vi "NameToData.vi"(11 "Name":string) -> (3 "Target":T1)   [LabVIEW 2018]
uses:
  TargetDataType.ctl
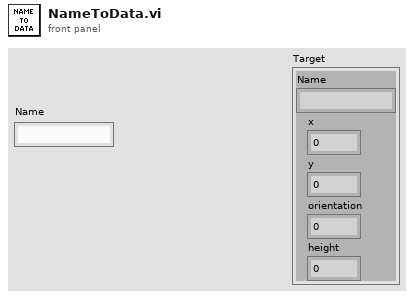
[diagram p1: front panel]
types:
  T1 = typedef "TargetDataType.ctl" = cluster{"Name":string, "x":dbl, "y":dbl, "orientation":dbl, "height":dbl}
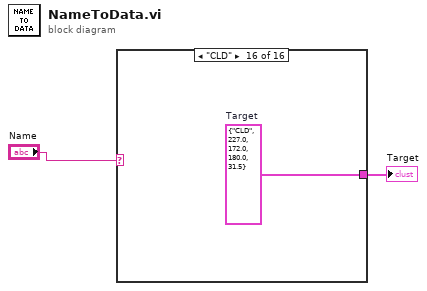
[diagram p0: block diagram]
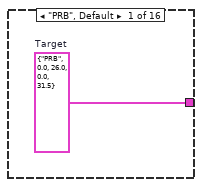
[diagram p2: hidden frame]
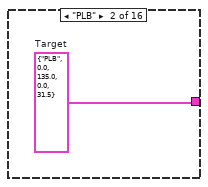
[diagram p3: hidden frame]
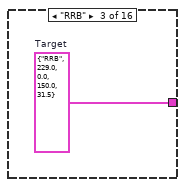
[diagram p4: hidden frame]
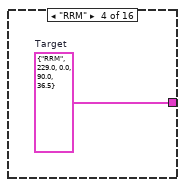
[diagram p5: hidden frame]
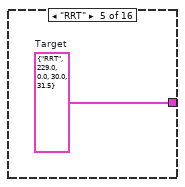
[diagram p6: hidden frame]
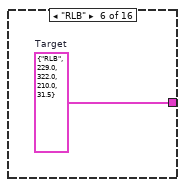
[diagram p7: hidden frame]
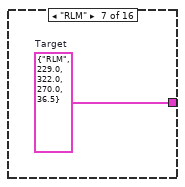
[diagram p8: hidden frame]
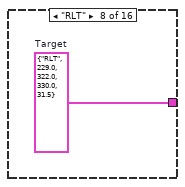
[diagram p9: hidden frame]
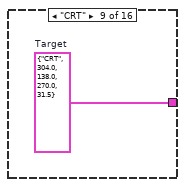
[diagram p10: hidden frame]
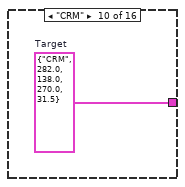
[diagram p11: hidden frame]
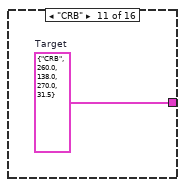
[diagram p12: hidden frame]
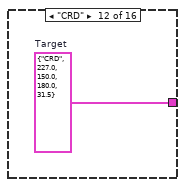
[diagram p13: hidden frame]
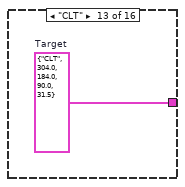
[diagram p14: hidden frame]
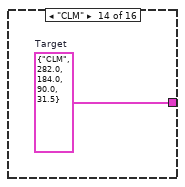
[diagram p15: hidden frame]
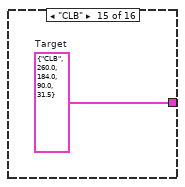
[diagram p16: hidden frame]
diagram:
  n1 = case shown="\"CLD\"" "Name" {
    tunnel: [w3 w4 w5 w6 w7 w8 w9 w10 w11 w12 w13 w14 w15 w16 w17 w18] -> w1
    frame "PRB", Default {
      w3 = T1 {"Name"="PRB", "x"=0.0, "y"=26.0, "orientation"=0.0, "height"=31.5}  # Target
    }
    frame "PLB" {
      w4 = T1 {"Name"="PLB", "x"=0.0, "y"=135.0, "orientation"=0.0, "height"=31.5}  # Target
    }
    frame "RRB" {
      w5 = T1 {"Name"="RRB", "x"=229.0, "y"=0.0, "orientation"=150.0, "height"=31.5}  # Target
    }
    frame "RRM" {
      w6 = T1 {"Name"="RRM", "x"=229.0, "y"=0.0, "orientation"=90.0, "height"=36.5}  # Target
    }
    frame "RRT" {
      w7 = T1 {"Name"="RRT", "x"=229.0, "y"=0.0, "orientation"=30.0, "height"=31.5}  # Target
    }
    frame "RLB" {
      w8 = T1 {"Name"="RLB", "x"=229.0, "y"=322.0, "orientation"=210.0, "height"=31.5}  # Target
    }
    frame "RLM" {
      w9 = T1 {"Name"="RLM", "x"=229.0, "y"=322.0, "orientation"=270.0, "height"=36.5}  # Target
    }
    frame "RLT" {
      w10 = T1 {"Name"="RLT", "x"=229.0, "y"=322.0, "orientation"=330.0, "height"=31.5}  # Target
    }
    frame "CRT" {
      w11 = T1 {"Name"="CRT", "x"=304.0, "y"=138.0, "orientation"=270.0, "height"=31.5}  # Target
    }
    frame "CRM" {
      w12 = T1 {"Name"="CRM", "x"=282.0, "y"=138.0, "orientation"=270.0, "height"=31.5}  # Target
    }
    frame "CRB" {
      w13 = T1 {"Name"="CRB", "x"=260.0, "y"=138.0, "orientation"=270.0, "height"=31.5}  # Target
    }
    frame "CRD" {
      w14 = T1 {"Name"="CRD", "x"=227.0, "y"=150.0, "orientation"=180.0, "height"=31.5}  # Target
    }
    frame "CLT" {
      w15 = T1 {"Name"="CLT", "x"=304.0, "y"=184.0, "orientation"=90.0, "height"=31.5}  # Target
    }
    frame "CLM" {
      w16 = T1 {"Name"="CLM", "x"=282.0, "y"=184.0, "orientation"=90.0, "height"=31.5}  # Target
    }
    frame "CLB" {
      w17 = T1 {"Name"="CLB", "x"=260.0, "y"=184.0, "orientation"=90.0, "height"=31.5}  # Target
    }
    frame "CLD" {
      w18 = T1 {"Name"="CLD", "x"=227.0, "y"=172.0, "orientation"=180.0, "height"=31.5}  # Target
    }
  }
  "Target" <- w1
